vi "Close.vi"(8 "error in":errorcluster, 11 "Overload Counter Channels in":refnum<class "Overload Counter Channels.lvclass">) -> (0 "error out":errorcluster, 3 "Overload Counter Channels out":refnum<class "Overload Counter Channels.lvclass">)   [LabVIEW 2023, in "Overload Counter Channels.lvclass"]
uses:
  Overload Counter Channels.lvclass
  <vilib>/ADAS Replay HIL/AdasHilServices/AdasHilChannelServices.lvlib
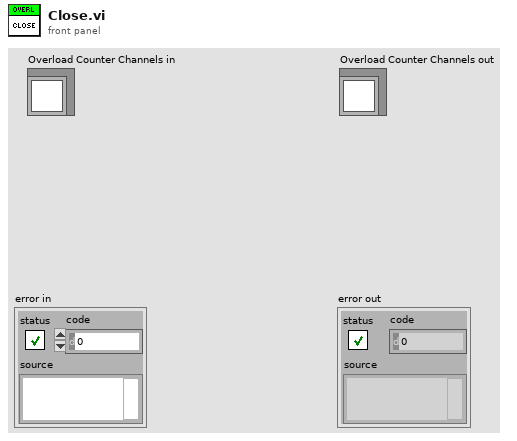
[diagram p1: front panel]
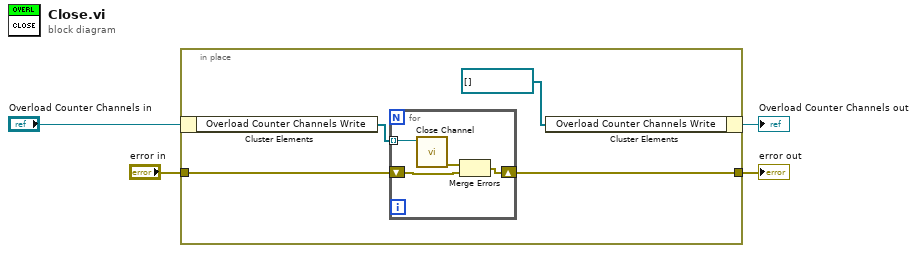
[diagram p0: block diagram]
diagram:
  n1 = in-place {
    in-place-border: "error in" -> [w8]
    in-place-border: [w7] -> w3
    n2 = in-place-cluster #1("Overload Counter Channels in") -> ("Overload Counter Channels Write"=w6:refnum<k21>[])
    n3 = for {
      tunnel: w6 -> [w12] mode=indexing
      shift-right: [w11] -> w7
      shift-left: w8 -> [w9]
      n4 = call <vilib>:"Close Channel.vi"("ADAS HIL Channel"=w12) -> ("error out"=w10:errorcluster)  [unwired: 10 in]
      n5 = Merge Errors(w10, w9) -> (w11:errorcluster)
    }
    n6 = in-place-cluster #1("Overload Counter Channels Write"=refnum<k21>[] [] ("Control Mode Read")) -> (→"Overload Counter Channels out":refnum<class "Overload Counter Channels.lvclass">)
  }
  "error out" <- w3
